vi "HP-get.vi"(7 "get byte count":u32, 8 "error in (no error)":errorcluster, 11 "HP-S-Serial in":refnum<class "HP-S-Serial.lvclass">) -> (0 "error out":errorcluster, 2 "read buffer":T1 format="%x", 3 "HP-S-Serial out":refnum<class "HP-S-Serial.lvclass">)   [LabVIEW 2020, in "HP-S-Serial.lvclass"]
uses:
  HP-S-Serial.lvclass
  HP-S-data.ctl
  HP-S-Serial.lvclass/HP-S-Serial.ctl
panel:
  out "length":i32
  out "size(s)":i32
  out "Serial Settings:Number of Bytes at Serial Port":u32
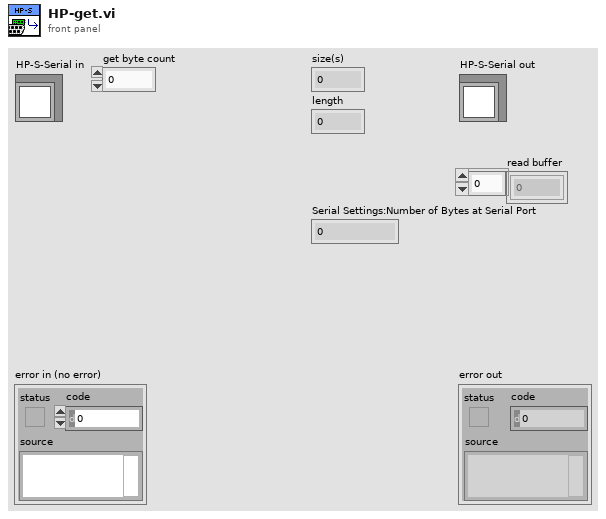
[diagram p1: front panel]
types:
  T1 = typedef "HP-S-Serial.lvclass/HP-S-data.ctl" = u8[]
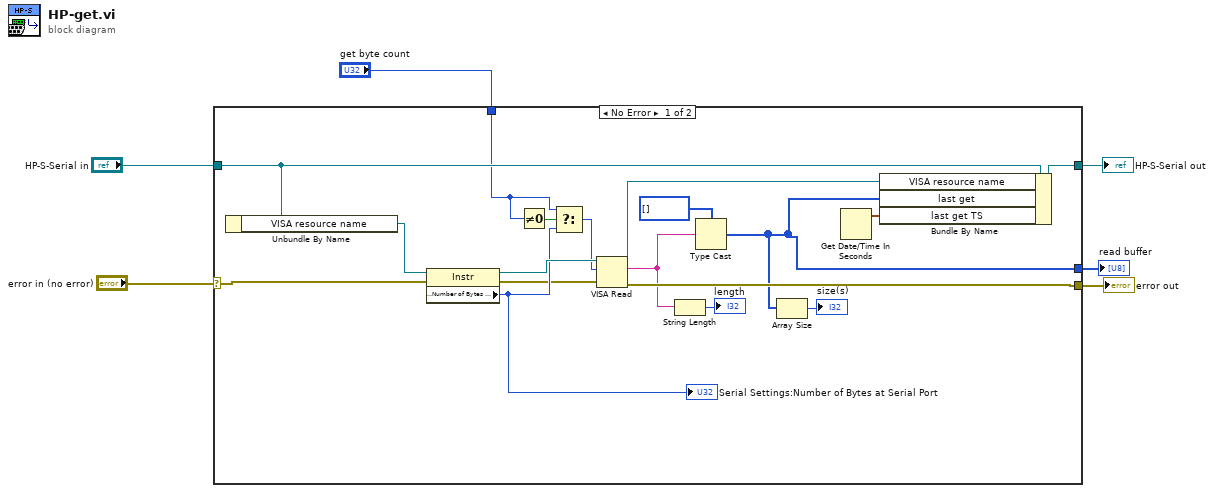
[diagram p0: block diagram]
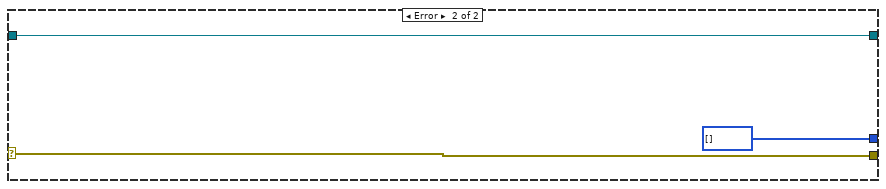
[diagram p2: hidden frame]
diagram:
  n1 = case shown="No Error" "error in (no error)" {
    selector: "error in (no error)" -> [w17 w27]
    tunnel: [w19 w27] -> w5
    tunnel: [w21 w26] -> w3
    tunnel: "HP-S-Serial in" -> [w24 w26]
    tunnel: [w14 T1 [] ("session.last get")] -> w2
    tunnel: "get byte count" -> [w10 _]
    frame No Error {
      n2 = Unbundle By Name(w24) -> ("VISA resource name"=w23:refnum<visa-resource-name>)
      n3 = property class="Instr"(reference=w23, error in=w17) -> (reference out=w22:refnum<visa-resource-name>, error out=w7:errorcluster, "Serial Settings:Number of Bytes at Serial Port"=w9:u32)
      "Serial Settings:Number of Bytes at Serial Port" <- w9
      n4 = Not Equal To 0?(x=w10) -> (x != 0?=w11:bool)
      n5 = Select(t=w10, s=w11, f=w9) -> (s? t:f=w8:u32)
      n6 = VISA Read(VISA resource name=w22, byte count=w8, error in (no error)=w7) -> (VISA resource name out=w20:refnum<visa-resource-name>, read buffer=w15:string, error out=w19:errorcluster)  [unwired: 1 out]
      n7 = String Length(string=w15) -> (length=→"length":i32)
      n8 = Type Cast(type=T1 [] ("read buffer"), x=w15) -> (*(type *) &x=w14:T1)
      n9 = Array Size(array=w14) -> (size(s)=→"size(s)":i32)
      n10 = Get Date/Time In Seconds() -> (seconds since 1Jan1904=w18:timestamp)
      n11 = Bundle By Name(cluster=w24, "VISA resource name"=w20, "last get"=w14, "last get TS"=w18) -> (w21:refnum<class "HP-S-Serial.lvclass">)
    }
    frame Error {
    }
  }
  "error out" <- w5
  "HP-S-Serial out" <- w3
  "read buffer" <- w2
